vi "PRL Insert Elements in String.vi"(10 "Elements":string[](array[string]), 11 "Input String":string) -> (3 "Output String":string)   [LabVIEW 2018, in "S3DK.lvlib" / "PMU Recorder Light.lvlib"]
uses:
  PMU Recorder Light.lvlib
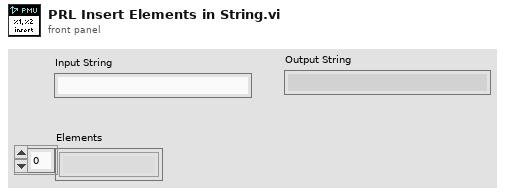
[diagram p1: front panel]
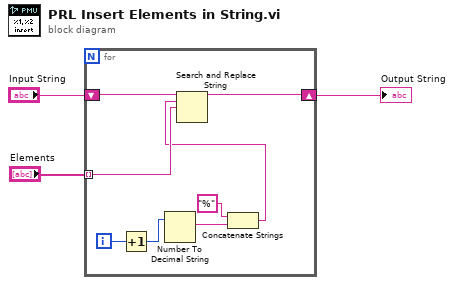
[diagram p0: block diagram]
diagram:
  n1 = for {
    shift-right: [w5] -> w3
    shift-left: "Input String" -> [w11]
    tunnel: "Elements" -> [w10] mode=indexing
    i -> [w9]
    n2 = Increment(x=w9) -> (x+1=w4:i32)
    n3 = Number To Decimal String(number=w4) -> (decimal integer string=w8:string)  [unwired: 1 out]
    n4 = Concatenate Strings("%" ("string"), w8) -> (w6:string)
    n5 = Search and Replace String(input string=w11, search string=w6, replace string=w10) -> (result string=w5:string)  [unwired: 1 in, 7 out]
  }
  "Output String" <- w3
